vi "MPVSenden-05-17.vi"(3 "Ventilposition":i32=1 min=1 max=6 step=1, 4 "error in":errorcluster, 5 "FPGA VI Reference In":refnum<k20>) -> (0 "Ventilposition":i32, 1 "error out":errorcluster, 2 "FPGA VI Reference Out":refnum<k20>)   [LabVIEW 2010]
uses:
  <vilib>/rvi/interface/nirviMethod/nirviMethod.xnode
  C:/Users/HAGAR-IV/Desktop/Zeugs/markus/version feb 2012/FPGA Bitfiles/pertrasgcfpga2_FPGATarget_FPGA-Programm-05_A75D3647.lvbitx
  C:/Users/HAGAR-IV/Desktop/Zeugs/Johnny/pertrasgc fpga/FPGA-Programm-05-17.vi
  <vilib>/rvi/interface/common/niFpgaNodeNameForErrorReporting.ctl
  <vilib>/rvi/errors/niLvFpgaWhatHappensToTopLevelVI.ctl
  GVVentilposition.vi
  <vilib>/Utility/error.llb/Error Cluster From Error Code.vi
  <vilib>/rvi/errors/niLvFpgaAdjustHostInterfaceError.vi
  NiFpgaLv.dll
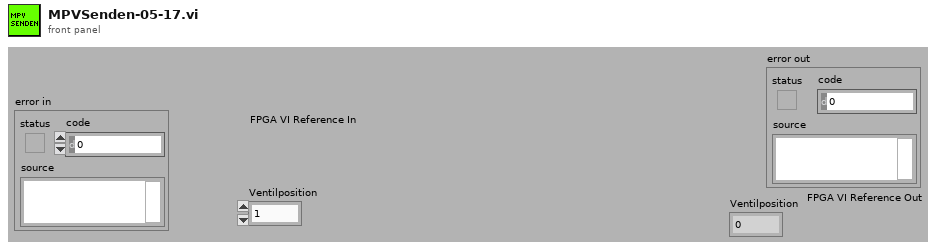
[diagram p1: front panel]
types:
  T1 = typedef "niFpgaNodeNameForErrorReporting.ctl" = enum16{"Open FPGA VI Reference", "Read/Write Control", "Invoke Method: Abort", "Invoke Method: Acknowledge IRQ", "Invoke Method: Download", "Invoke Method: FIFO.Configure", "Invoke Method: FIFO.Read", "Invoke Method: FIFO.Start", "Invoke Method: FIFO.Stop", "Invoke Method: FIFO.Write", "Invoke Method: Reset", "Invoke Method: Run", "Invoke Method: Wait on IRQ", "Close FPGA VI Reference"}
  T2 = typedef "niLvFpgaWhatHappensToTopLevelVI.ctl" = enum16{"top level VI scripted behind XNode", "top level VI inlined behind XNode"}
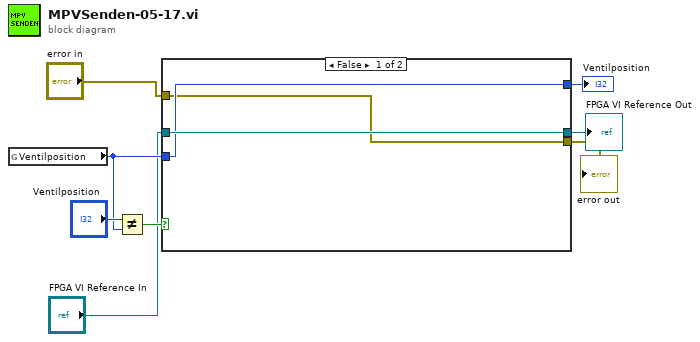
[diagram p0: block diagram]
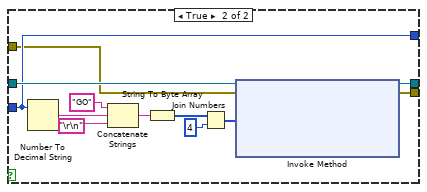
[diagram p2: hidden frame]
diagram:
  n1 = global read "GVVentilposition.vi" "Ventilposition"() -> (w6:i32)
  n2 = Not Equal?(x="Ventilposition", y=w6) -> (x != y?=w7:bool)
  n3 = case shown="False" w7 {
    tunnel: "FPGA VI Reference In" -> [w11 w23]
    tunnel: [w11 w15] -> w1
    tunnel: w6 -> [w10 w14]
    tunnel: [w10 w14] -> w5
    tunnel: "error in" -> [w9 w13]
    tunnel: [w9 w12] -> w3
    frame False {
    }
    frame True {
      n4 = Number To Decimal String(number=w14) -> (decimal integer string=w16:string)  [unwired: 1 in]
      n5 = Concatenate Strings("GO", w16, "\r\n") -> (w21:string)
      n6 = String To Byte Array(string=w21) -> (unsigned byte array=w20:u8[])
      n7 = Join Numbers(hi=w20, lo=u8 4) -> ((hi.lo)=w18:u16[])
      n8 = xnode "Invoke Method"("FPGA VI Reference In"=w23, "error in"=w13, "Data"=w18) -> ("FPGA VI Reference Out"=w15:refnum<k20>, "error out"=w12:errorcluster)  [unwired: 1 in, 1 out]
    }
  }
  "Ventilposition" <- w5
  "error out" <- w3
  "FPGA VI Reference Out" <- w1
